vi "主画面.vi"() -> ()   [LabVIEW 2016]
uses:
  <vilib>/Utility/sysdir.llb/System Directory Type.ctl
  <vilib>/NI/Modbus Library/API/Wrapper/Create TCP Slave.vi
  <vilib>/Utility/config.llb/Write Key (String).vi
  <vilib>/NI/Modbus Library/API/slave/Modbus Slave.lvclass
  <vilib>/Utility/config.llb/NI_LVConfig.lvlib
  data/FreeMem.dll
  <vilib>/NI/Modbus Library/API/Wrapper/API Main.lvlib
panel:
  out "error out":errorcluster caption="错误输出"
  in  "error in (no error)":errorcluster caption="错误输入（无错误）"
  out "字符串":string
  in  "全屏":T1
  out "站点名称":string="站点名称"
  out "时间显示":string="2017-05-09 10:50:42"
  out "Version":string="Version:1.0.0"
  in  "主画面菜单":enum32{"首页", "数据查询", "运维调试", "系统设置"}(xcontrol)
  # "ESTD-XP 一体化水质自动监测系统"
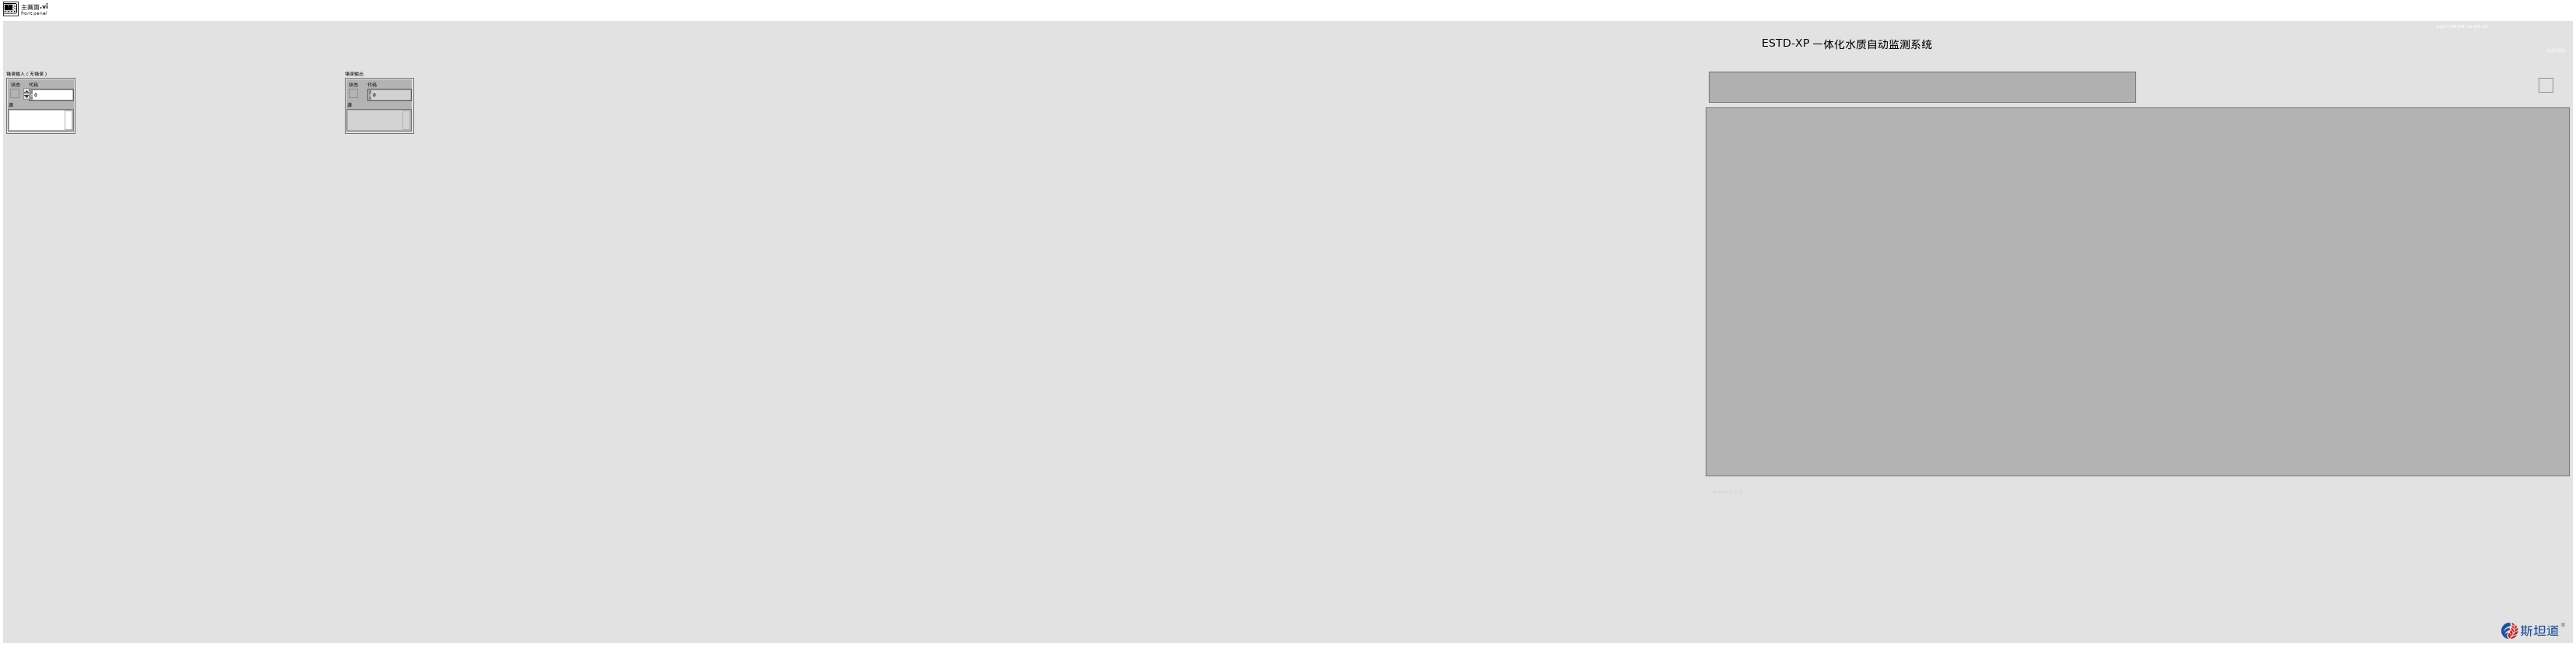
[diagram p1: front panel]
types:
  T1 = typedef "全屏按钮.ctl" = bool
  T2 = typedef "System Directory Type.ctl" = i32
  T3 = cluster{"时间标识":timestamp, "设备":string, "日志信息":string, "流程参数":string}
  T4 = enum32{"invalid app kind", "Development System", "Run Time System", "Student Edition", "Embedded LabVIEW", "Evaluation", "Custom"}
  T5 = enum32{"Bad", "Idle", "Run top level", "Running"}
  T6 = typedef "NI_LVConfig.lvlib/Config Data RefNum.ctl" = refnum<k1>
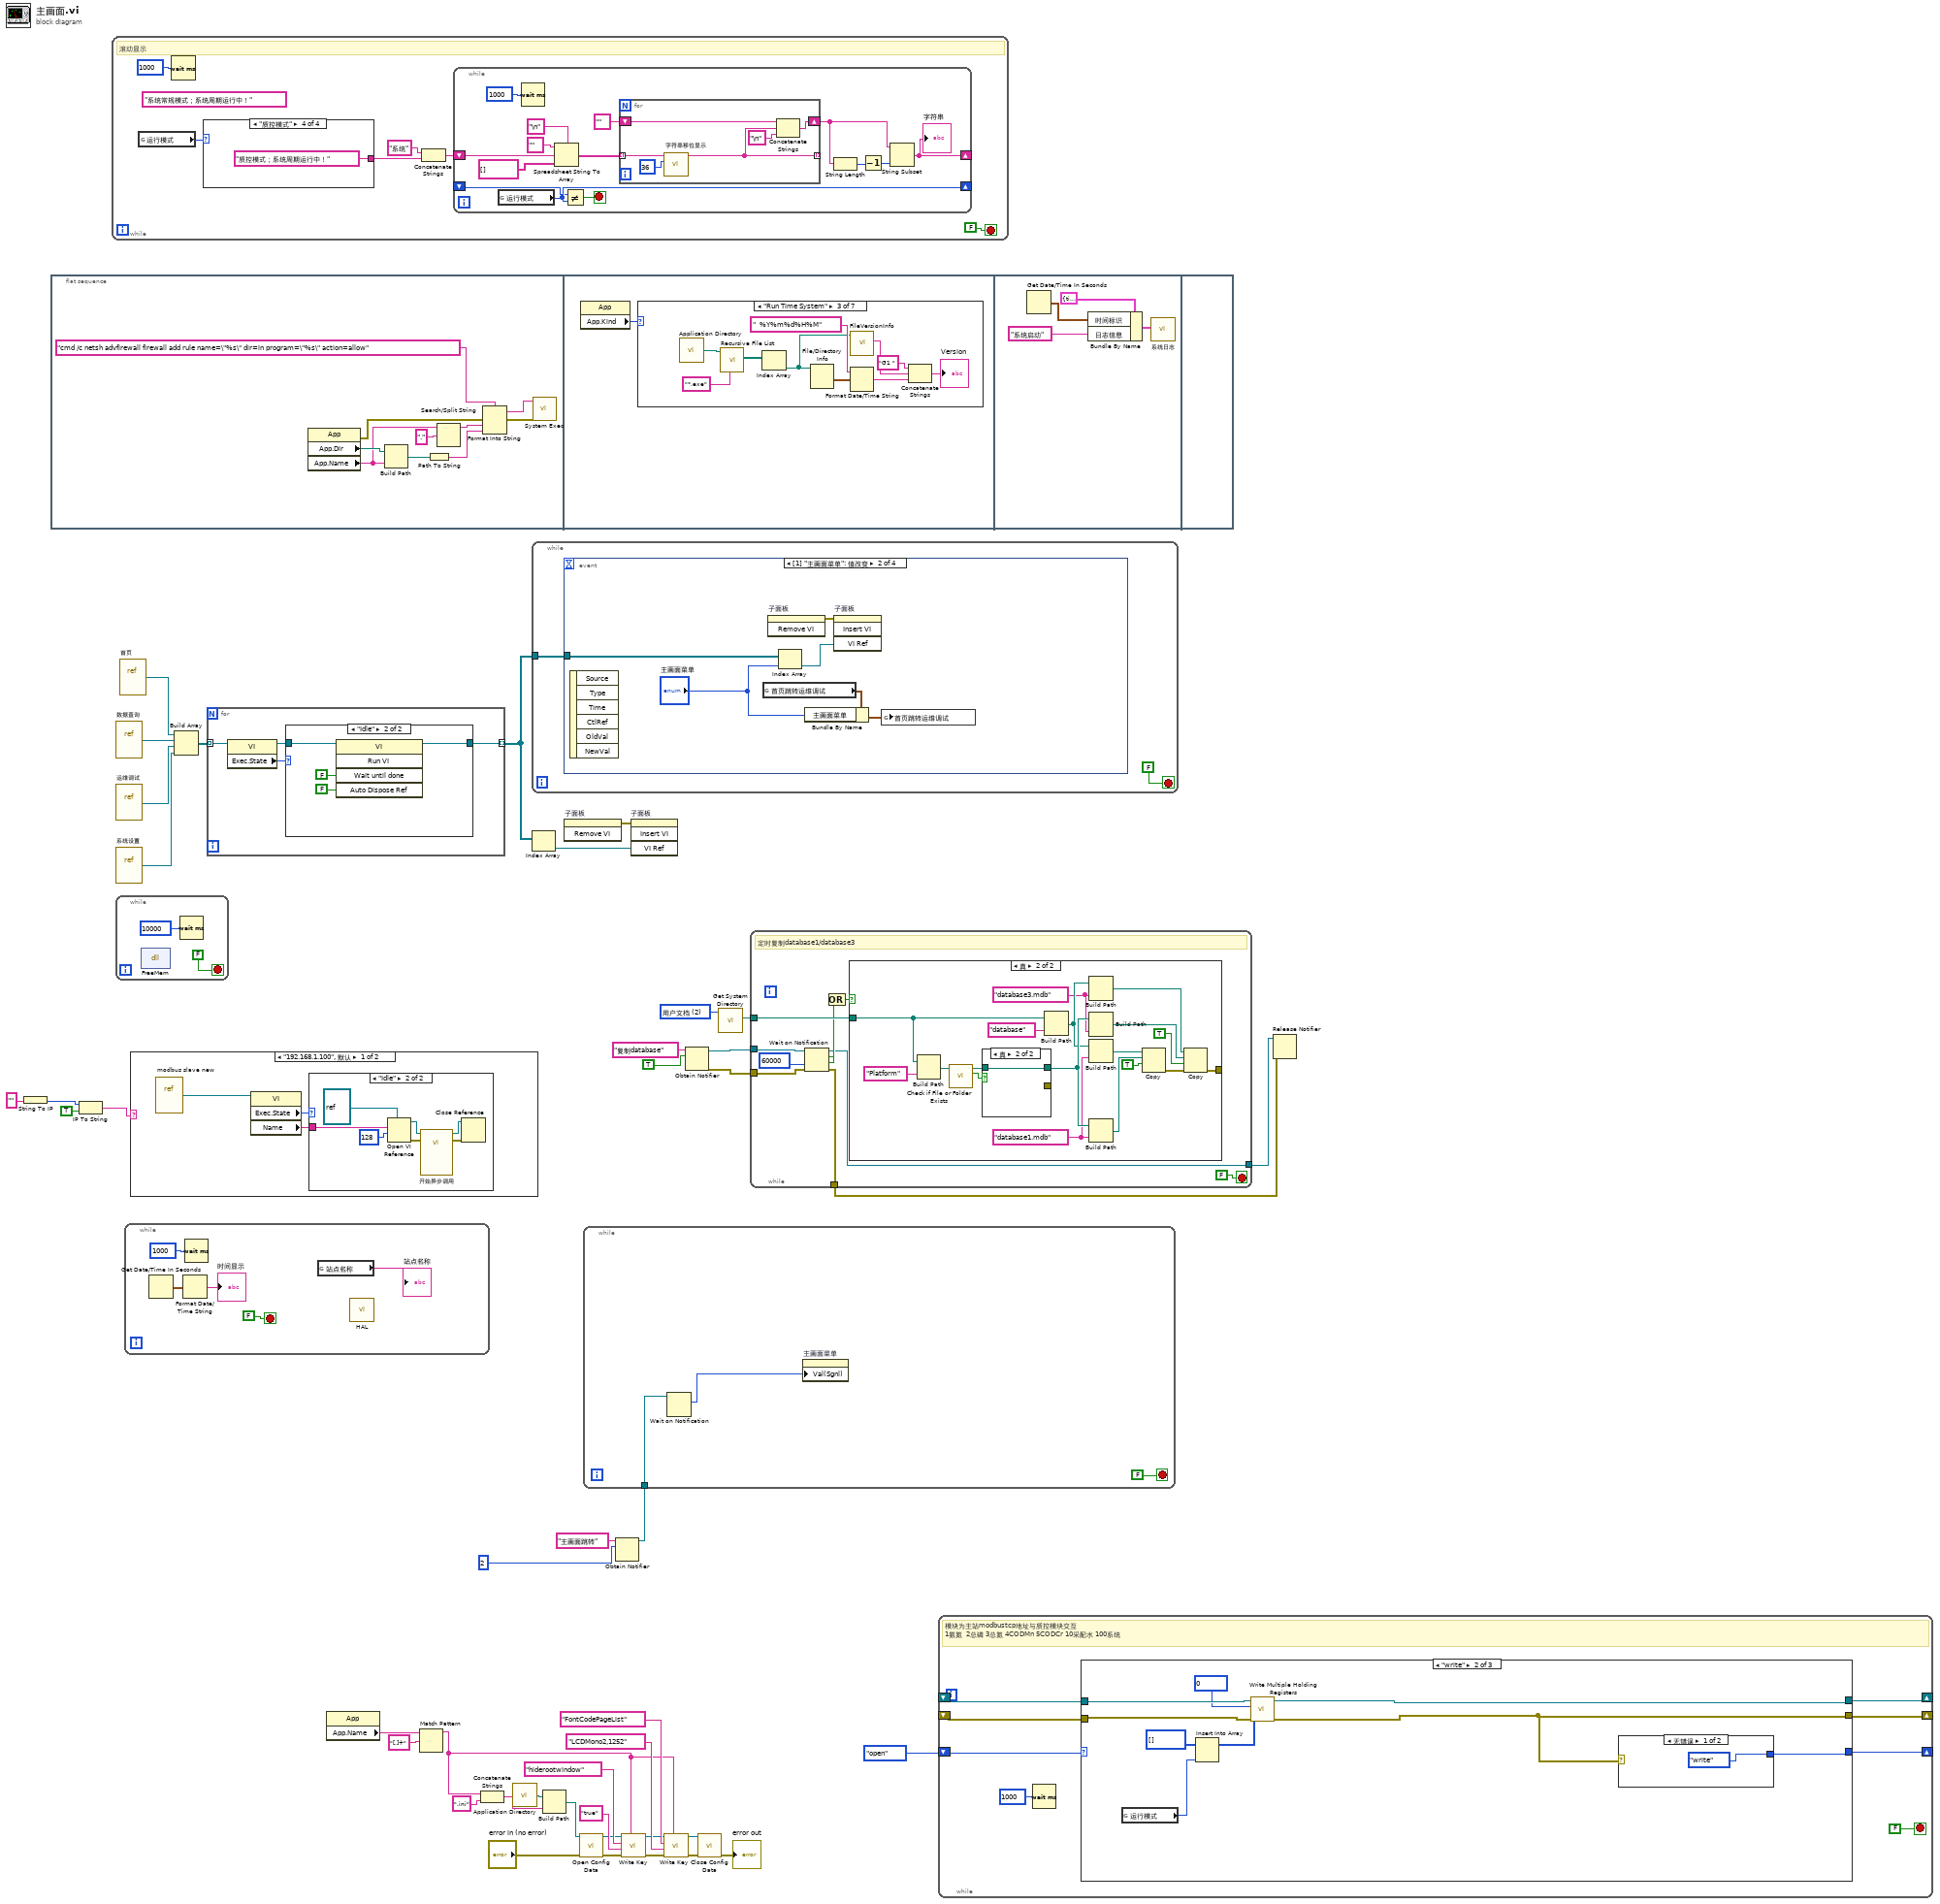
[diagram p0: block diagram]
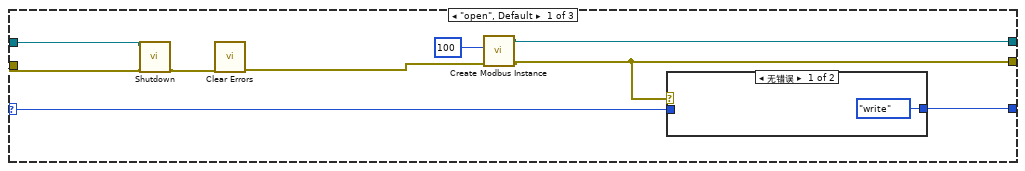
[diagram p2: hidden frame]
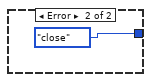
[diagram p4: hidden frame]
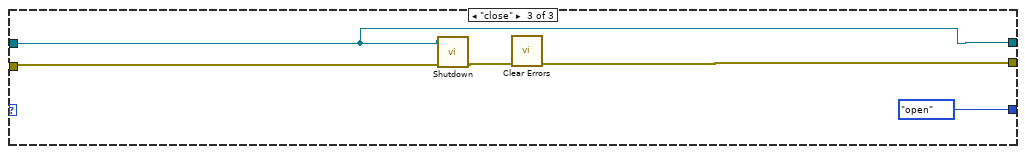
[diagram p5: hidden frame]
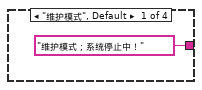
[diagram p6: hidden frame]
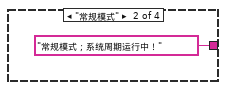
[diagram p7: hidden frame]
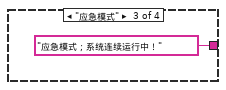
[diagram p8: hidden frame]
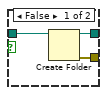
[diagram p12: hidden frame]
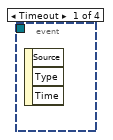
[diagram p20: hidden frame]
diagram:
  w35 = T2 2 items=["用户目录"=0, "用户桌面"=1, "用户文档"=2, "用户应用程序数据"=3, "用户设置"=4, "用户临时目录"=5, "公共文档"=6, "公共应用程序数据"=7, "公共设置"=8, "公共缓存"=13, "系统核心库"=9, "系统安装库"=10, "应用程序文件"=11, "启动盘根目录"=12] ("system directory type")
  n1 = String To IP(1:"" ("名称")) -> (0:w33:u32)
  n2 = flat-sequence {
    frame #0 {
      n3 = property class="App"() -> (error out=w45:errorcluster, "App.Dir"=w53:path, "App.Name"=w48:string)  [unwired: 2 in, 1 out]
      n4 = Build Path(base path=w53, name or relative path=w48) -> (appended path=w52:path)
      n5 = Path To String(path=w52) -> (string=w50:string)
      n6 = Search/Split String(string=w48, search string/char (-)="." ("搜索字符串/字符(-)")) -> (substring before match=w47:string)  [unwired: 1 in, 2 out]
      n7 = Format Into String(format string="cmd /c netsh advfirewall firewall add rule name=\"%s\" dir=in program=\"%s\" action=allow" ("command line"), error in=w45, w47, w50) -> (resulting string=w46:string, error out=w44:errorcluster)  [unwired: 1 in]
      n8 = call <vilib>:"System Exec.vi"("error in (no error)"=w44, "command line"=w46) -> ()  [unwired: 6 in, 4 out]
    }
    frame #1 {
      n9 = property class="App"() -> ("App.Kind"=w54:T4)  [unwired: 2 in, 2 out]
      n10 = case shown="\"Run Time System\"" w54 {
        frame "invalid app kind" {
        }
        frame "Development System", Default {
        }
        frame "Run Time System" {
          n11 = call <vilib>:"Application Directory.vi"() -> ("Application Directory"=w57:path)
          n12 = call <vilib>:"Recursive File List.vi"("pattern"="*.exe", "Folder Path"=w57) -> ("All Files in Dir"=w58:path[])  [unwired: 5 in, 4 out]
          n13 = Index Array(array=w58) -> (element=w56:path)  [unwired: 1 in]
          n14 = File/Directory Info(path=w56) -> (last mod=w62:timestamp)  [unwired: 1 in, 6 out]
          n15 = call <vilib>:"FileVersionInfo.vi"("Application Path in"=w56) -> ("File Version Info"=w55:string)  [unwired: 7 in, 3 out]
          n16 = Format Date/Time String(time format string (%c)="  %Y%m%d%H%M" ("时间格式字符串(%c)"), seconds (now)=w62) -> (date/time string=w60:string)  [unwired: 1 in]
          n17 = Concatenate Strings("G1 " ("字符串"), w55, w60) -> (→"Version":string)
        }
        frame "Student Edition" {
        }
        frame "Embedded LabVIEW" {
        }
        frame "Evaluation" {
        }
        frame "Custom" {
        }
      }
    }
    frame #2 {
      n18 = Get Date/Time In Seconds() -> (seconds since 1Jan1904=w66:timestamp)
      n19 = Bundle By Name(cluster=T3 {"时间标识"=timestamp(0 s since 1904-01-01), "设备"="系统", "日志信息"="", "流程参数"=""} ("data in"), "时间标识"=w66, "日志信息"="系统启动") -> (w67:T3)
      n20 = call "系统日志.vi"("data in"=w67) -> ()  [unwired: 11 in]
    }
    frame #3 {
    }
  }
  n21 = IP To String(1:TRUE ("句点符号？(F)"), 2:w33) -> (0:w30:string)
  n22 = while {
    stop <- FALSE stop-if-true
    (unwired) "系统常规模式；系统周期运行中！" ("字符串")
    # "滚动显示"
    n23 = global read "系统设置全局变量.vi" "运行模式"() -> (w71:enum16{"维护模式", "常规模式", "应急模式", "质控模式"})
    n24 = Wait (ms)(milliseconds to wait=u32 1000 ("等待时间（毫秒）")) -> ()  [unwired: 1 out]
    n25 = case shown="\"质控模式\"" w71 {
      tunnel: ["维护模式；系统停止中！" "常规模式；系统周期运行中！" "应急模式；系统连续运行中！" "质控模式；系统周期运行中！"] -> w70
      frame "维护模式", Default {
      }
      frame "常规模式" {
      }
      frame "应急模式" {
      }
      frame "质控模式" {
      }
    }
    n26 = Concatenate Strings("系统" ("字符串"), w70) -> (w69:string)
    n27 = while {
      shift-right: [w82] -> _
      shift-left: w69 -> [w87]
      shift-right: [w81] -> _
      shift-left: _ -> [w80]
      stop <- w79 stop-if-true
      n28 = global read "系统设置全局变量.vi" "运行模式"() -> (w81:enum16{"维护模式", "常规模式", "应急模式", "质控模式"})
      n29 = Wait (ms)(milliseconds to wait=u32 1000 ("等待时间（毫秒）")) -> ()  [unwired: 1 out]
      n30 = Spreadsheet String To Array(delimiter (Tab)="\n" ("分隔符(Tab)"), format string="" ("格式字符串"), spreadsheet string=w87, array type (2D Dbl)=string[] []) -> (array=w90:string[])
      n31 = Not Equal?(x=w80, y=w81) -> (x != y?=w79:bool)
      n32 = for {
        tunnel: w90 -> [w98] mode=indexing
        tunnel: [w96] -> _ mode=indexing
        shift-right: [w94] -> w85
        shift-left: "" ("格式字符串") -> [w95]
        n33 = call "字符串移位显示.vi"("字符框大小"=36, "字符串输入"=w98) -> ("移位后字符串"=w96:string)  [unwired: 8 in, 1 out]
        n34 = Concatenate Strings(w95, w96, "\n" ("分隔符(Tab)")) -> (w94:string)
      }
      n35 = String Length(string=w85) -> (length=w84:i32)
      n36 = Decrement(x=w84) -> (x-1=w83:i32)
      n37 = String Subset(string=w85, length (rest)=w83) -> (substring=w82:string)  [unwired: 1 in]
      "字符串" <- w82
    }
  }
  n38 = vi-ref "数据查询.vi"() -> (w39:refnum<vi>)
  n39 = vi-ref "运维调试.vi"() -> (w38:refnum<vi>)
  n40 = vi-ref "系统设置.vi"() -> (w37:refnum<vi>)
  n41 = while {
    stop <- FALSE stop-if-true
    n42 = dll-call lib="PTH2qabs CUsersHsiao\tDocumentsGIT\t固定站,一体站项目 - 固定站模板 - 新CODMndataFreeMem.dll" fn="FreeMem"() -> ()  [unwired: 4 in, 2 out]
    n43 = Wait (ms)(milliseconds to wait=u32 10000 ("等待时间（毫秒）")) -> ()  [unwired: 1 out]
  }
  n44 = vi-ref "首页.vi"() -> (w40:refnum<vi>)
  n45 = while {
    stop <- FALSE stop-if-true
    n46 = Get Date/Time In Seconds() -> (seconds since 1Jan1904=w102:timestamp)
    n47 = Format Date/Time String(seconds (now)=w102) -> (date/time string=→"时间显示":string)  [unwired: 2 in]
    n48 = Wait (ms)(milliseconds to wait=u32 1000 ("等待时间（毫秒）")) -> ()  [unwired: 1 out]
    n49 = global read "系统设置全局变量.vi" "站点名称"() -> (→"站点名称":string)
    n50 = call "HAL.vi"() -> ()  [unwired: 12 in]
  }
  n51 = case shown="\"192.168.1.100\", 默认" w30 {
    frame "192.168.1.100", Default {
      n52 = vi-ref "modbus slave new.vi"() -> (w106:refnum<vi>)
      n53 = property class="VI"(reference=w106) -> ("Exec.State"=w107:T5, "Name"=w108:string)  [unwired: 1 in, 2 out]
      n54 = case shown="\"Idle\"" w107 {
        tunnel: w108 -> [_ w109]
        frame "Bad", Default {
        }
        frame "Idle" {
          n55 = Open VI Reference(type specifier VI Refnum (for type only)=refnum<vi> refnum, vi path=w109, options=128 ("选项")) -> (vi reference=w111:refnum<vi>, error out=w114:errorcluster)  [unwired: 3 in]
          n56 = call-by-ref "开始异步调用"(reference=w111, error in=w114) -> (reference out=w113:refnum<vi>, error out=w115:errorcluster)  [unwired: 12 in]
          n57 = Close Reference(reference=w113, error in (no error)=w115) -> ()  [unwired: 1 out]
        }
      }
    }
    frame "192.168.1.101" {
    }
  }
  n58 = Build Array(w40, w39, w38, w37) -> (w36:refnum<vi>[])
  n59 = for {
    tunnel: w36 -> [w119] mode=indexing
    tunnel: [w116] -> w42 mode=indexing
    n60 = property class="VI"(reference=w119) -> (reference out=w117:refnum<vi>, "Exec.State"=w118:T5)  [unwired: 1 in, 1 out]
    n61 = case shown="\"Idle\"" w118 {
      tunnel: w117 -> [w120 w122]
      tunnel: [w120 w121] -> w116
      frame "Bad", Default {
      }
      frame "Idle" {
        n62 = invoke class="VI" method="Run VI"(reference=w122, "Wait until done"=FALSE ("结束前等待"), "Auto Dispose Ref"=FALSE ("自动销毁引用")) -> (reference out=w121:refnum<vi>)  [unwired: 2 in, 4 out]
      }
    }
  }
  n63 = property class="App"() -> ("App.Name"=w13:string)  [unwired: 2 in, 2 out]
  n64 = Match Pattern(string=w13, regular expression="[.]+" ("正则表达式")) -> (before substring=w22:string)  [unwired: 1 in, 3 out]
  n65 = Concatenate Strings(w22, ".ini" ("字符串")) -> (w9:string)
  n66 = call <vilib>:"Application Directory.vi"() -> ("Application Directory"=w12:path)
  n67 = while {
    tunnel: w42 -> [w125]
    stop <- FALSE stop-if-true
    n68 = event shown="[1] \"主画面菜单\": 值改变" {
      selector: _ -> [_ _ _ _]
      dyn-events: _ -> [_ _ _ _]
      timeout: _ -> [_ _ _ _]
      tunnel: w125 -> [_ w132 _ _]
      event Timeout {
        n69 = event-data() -> ()  [unwired: 1 in, 3 out]
      }
      event "主画面菜单": Value Change {
        n70 = event-data() -> ()  [unwired: 1 in, 6 out]
        n71 = global read "系统设置全局变量.vi" "首页跳转运维调试"() -> (w129:cluster{"主画面菜单":i32, "运维调试菜单":i32})
        n72 = invoke on="子面板" class="SubPnl" method="Remove VI"() -> (error out=w130:errorcluster)  [unwired: 3 in, 2 out]
        n73 = Index Array(array=w132, index="主画面菜单") -> (element=w131:refnum<vi>)
        n74 = Bundle By Name(cluster=w129, "主画面菜单"="主画面菜单") -> (w128:cluster{"主画面菜单":i32, "运维调试菜单":i32})
        n75 = invoke on="子面板" class="SubPnl" method="Insert VI"(error in=w130, "VI Ref"=w131) -> ()  [unwired: 2 in, 4 out]
        n76 = global write "系统设置全局变量.vi" "首页跳转运维调试"(w128) -> ()
      }
      event Panel Close? {
        n77 = event-data() -> ()  [unwired: 1 in, 4 out]
        n78 = flat-sequence {
          frame #0 {
            n79 = Get Date/Time In Seconds() -> (seconds since 1Jan1904=w136:timestamp)
            n80 = Bundle By Name(cluster=T3 {"时间标识"=timestamp(0 s since 1904-01-01), "设备"="系统", "日志信息"="", "流程参数"=""} ("data in"), "时间标识"=w136, "日志信息"="系统关闭") -> (w135:T3)
            n81 = call "系统日志.vi"("data in"=w135) -> ()  [unwired: 11 in]
          }
          frame #1 {
            n82 = call "Force Quit LabVIEW.vi"() -> ()  [unwired: 10 in, 2 out]
          }
          frame #2 {
            n83 = Quit LabVIEW(quit? (T)=TRUE ("退出？(T)")) -> ()
          }
        }
        n84 = event-data("Discard?"=FALSE ("放弃？")) -> ()  [unwired: 1 in, 1 out]
      }
      event Value Change {
        n85 = event-data() -> ("NewVal"=w142:T1)  [unwired: 1 in, 5 out]
        n86 = case shown="真" w142 {
          tunnel: [1920 ("Panel Width") 1600 ("Panel Width")] -> w141
          tunnel: [1080 ("Panel Height") 900 ("Panel Height")] -> w140
          frame False {
          }
          frame True {
          }
        }
        n87 = control-ref of="本VI"() -> (w147:refnum<vi>)
        n88 = property class="VI"(reference=w147, "Front Panel.TitleBarVis"=w142, "Front Panel.IsFrontmost"=TRUE ("前面板窗口:在最前")) -> (reference out=w143:refnum<vi>)  [unwired: 1 in, 1 out]
        n89 = Close Reference(reference=w143) -> ()  [unwired: 1 in, 1 out]
        n90 = Current VI's Path() -> (path=w146:path)
        n91 = call "Set panel size and  place center.vi"("Path"=w146, "Close Reference (false)"=TRUE, "Panel Width"=w141, "Panel Height"=w140, "FP.Origin in(H & V)"=cluster{"Horizontal":i16, "Vertical":i16} {"Horizontal"=0, "Vertical"=0}) -> ()  [unwired: 6 in, 5 out]
      }
    }
  }
  n92 = Index Array(array=w42) -> (element=w41:refnum<vi>)  [unwired: 1 in]
  n93 = Build Path(base path=w12, name or relative path=w9) -> (appended path=w15:path)
  n94 = invoke on="子面板" class="SubPnl" method="Remove VI"() -> (error out=w43:errorcluster)  [unwired: 3 in, 2 out]
  n95 = call <vilib>:"Open Config Data.vi"("error in (no error)"="error in (no error)", "configuration file path"=w15) -> ("error out"=w17:errorcluster, "refnum"=w16:T6)  [unwired: 7 in, 1 out]
  n96 = Obtain Notifier(name (unnamed)="主画面跳转" ("名称（未命名）"), notification data type=2 ("主画面菜单")) -> (notifier out=w28:refnum<notifier>)  [unwired: 2 in, 2 out]
  n97 = while {
    tunnel: w28 -> [w153]
    stop <- FALSE stop-if-true
    n98 = Wait on Notification(notifier=w153) -> (notification=w152:i32)  [unwired: 3 in, 3 out]
    n99 = property on="主画面菜单" class="主画面菜单 (严格)"("Val(Sgnl)"=w152) -> ()  [unwired: 2 in, 2 out]
  }
  n100 = call-poly <vilib>:"Write Key.vi"("section"=w22, "error in (no error)"=w17, "value"="true" ("key"), "key"="hiderootwindow", "refnum"=w16) -> ("error out"=w20:errorcluster, "refnum out"=w21:T6)  [unwired: 4 in, 1 out]
  n101 = invoke on="子面板" class="SubPnl" method="Insert VI"(error in=w43, "VI Ref"=w41) -> ()  [unwired: 2 in, 4 out]
  n102 = call-poly <vilib>:"Write Key.vi"("section"=w22, "error in (no error)"=w20, "value"="LCDMono2,1252" ("key"), "key"="FontCodePageList", "refnum"=w21) -> ("error out"=w25:errorcluster, "refnum out"=w26:T6)  [unwired: 4 in, 1 out]
  n103 = Obtain Notifier(name (unnamed)="复制database" ("名称（未命名）"), notification data type=TRUE) -> (notifier out=w7:refnum<notifier>, error out=w6:errorcluster)  [unwired: 2 in, 1 out]
  n104 = call <vilib>:"Close Config Data.vi"("error in (no error)"=w25, "refnum"=w26) -> ("error out"=→"error out":errorcluster)  [unwired: 8 in, 1 out]
  n105 = call <vilib>:"Get System Directory.vi"("system directory type"=w35) -> ("system directory"=w34:path)  [unwired: 10 in]
  n106 = while {
    tunnel: w34 -> [w163]
    tunnel: w7 -> [w161]
    tunnel: w6 -> [w160]
    tunnel: [w156] -> w3
    tunnel: [w155] -> w2
    stop <- FALSE stop-if-true
    # "定时复制database1/database3"
    n107 = Wait on Notification(notifier=w161, timeout in ms (-1)=60000 ("超时毫秒(-1)"), error in (no error)=w160) -> (notifier out=w156:refnum<notifier>, notification=w158:bool, timed out?=w159:bool, error out=w155:errorcluster)  [unwired: 1 in]
    n108 = Or(x=w158, y=w159) -> (x .or. y?=w157:bool)
    n109 = case shown="真" w157 {
      tunnel: w163 -> [_ w172]
      tunnel: [_ w168] -> _
      frame False {
      }
      frame True {
        w166 = "database1.mdb" ("名称或相对路径")
        w167 = "database3.mdb" ("名称或相对路径")
        n110 = Build Path(base path=w172, name or relative path="Platform" ("名称或相对路径")) -> (appended path=w179:path)
        n111 = call <vilib>:"Check if File or Folder Exists.vi"("path"=w179) -> ("file or folder exists?"=w178:bool, "dup path"=w177:path)  [unwired: 8 in, 1 out]
        n112 = case shown="真" w178 {
          tunnel: [w184 w186] -> w174
          tunnel: w177 -> [w185 w186]
          tunnel: [w183 _] -> _
          frame False {
            n113 = Create Folder(path (use dialog)=w185) -> (created path=w184:path, error out=w183:errorcluster)  [unwired: 2 in, 1 out]
          }
          frame True {
          }
        }
        n114 = Build Path(base path=w172, name or relative path="database" ("名称或相对路径")) -> (appended path=w170:path)
        n115 = Build Path(base path=w170, name or relative path=w167) -> (appended path=w169:path)
        n116 = Build Path(base path=w174, name or relative path=w167) -> (appended path=w173:path)
        n117 = Build Path(base path=w170, name or relative path=w166) -> (appended path=w171:path)
        n118 = Build Path(base path=w174, name or relative path=w166) -> (appended path=w176:path)
        n119 = Copy(9:TRUE ("覆盖(F)"), 10:w176, 11:w171) -> (0:w175:errorcluster)  [unwired: 2 in, 2 out]
        n120 = Copy(8:w175, 9:TRUE ("覆盖(F)"), 10:w173, 11:w169) -> (0:w168:errorcluster)  [unwired: 1 in, 2 out]
      }
    }
  }
  n121 = while {
    shift-right: [w192] -> _
    shift-left: _ -> [w194]
    shift-right: [w191] -> _
    shift-left: _ -> [w193]
    shift-right: [w188] -> _
    shift-left: enum16{"open", "read", "write", "close"}."open" -> [w189]
    stop <- FALSE stop-if-true
    # "模块为主站modbustcp地址与质控模块交互\n1氨氮  2总磷 3总氮 4CODMn 5CODCr 10采配水 100系统"
    n122 = Wait (ms)(milliseconds to wait=u32 1000 ("等待时间（毫秒）")) -> ()  [unwired: 1 out]
    n123 = case shown="\"write\"" w189 {
      selector: w189 -> [w203 _ _]
      tunnel: w194 -> [w197 w213 w219]
      tunnel: w193 -> [w196 w212 w218]
      tunnel: [w200 w207 w219] -> w192
      tunnel: [w199 w206 w221] -> w191
      tunnel: [w202 w214 enum16{"open", "read", "write", "close"}."open"] -> w188
      frame "open", Default {
        n124 = call-dynamic "Shutdown.vi"("error in"=w196, "Modbus slave in"=w197) -> ("error out"=w195:errorcluster)  [unwired: 9 in]
        n125 = call <vilib>:"Clear Errors.vi"("error in (no error)"=w195) -> ("error out"=w198:errorcluster)  [unwired: 5 in, 1 out]
        n126 = call-poly <vilib>:"Create Modbus Instance.vi"("error in"=w198, "port (502)"=u16 100) -> ("error out"=w199:errorcluster, "TCP slave instance"=w200:refnum<class "Modbus Slave.lvclass">)  [unwired: 8 in]
        n127 = case shown="无错误" w199 {
          tunnel: w203 -> [_ w205]
          tunnel: [enum16{"open", "read", "write", "close"}."write" w205] -> w202
          frame No Error {
          }
          frame Error {
          }
        }
      }
      frame "write" {
        n128 = global read "系统设置全局变量.vi" "运行模式"() -> (w209:enum16{"维护模式", "常规模式", "应急模式", "质控模式"})
        n129 = Insert Into Array(array=u16[] [] ("registers to write"), new element=w209) -> (w208:u16[])  [unwired: 1 in]
        n130 = call-dynamic "Write Multiple Holding Registers.vi"("error in"=w212, "registers to write"=w208, "starting address"=u16 0, "Modbus slave in"=w213) -> ("error out"=w206:errorcluster, "Modbus slave out"=w207:refnum<class "Modbus Slave.lvclass">)  [unwired: 6 in]
        n131 = case shown="无错误" w206 {
          tunnel: [enum16{"open", "read", "write", "close"}."write" enum16{"open", "read", "write", "close"}."close"] -> w214
          frame No Error {
          }
          frame Error {
          }
        }
      }
      frame "close" {
        n132 = call-dynamic "Shutdown.vi"("error in"=w218, "Modbus slave in"=w219) -> ("error out"=w217:errorcluster)  [unwired: 9 in]
        n133 = call <vilib>:"Clear Errors.vi"("error in (no error)"=w217) -> ("error out"=w221:errorcluster)  [unwired: 5 in, 1 out]
      }
    }
  }
  n134 = Release Notifier(notifier=w3, error in (no error)=w2) -> ()  [unwired: 1 in, 3 out]
